vi "CF_FP_to_DSC.vi"(8 "error in (no error)":errorcluster, 10 "str":string[](array[string]), 11 "dbl":dbl[](array[numeric])) -> (0 "error out":errorcluster)   [LabVIEW 2016]
panel:
  in  "str var":refnum<k21>[](array[refnum])=["ni.var.psp://housesoftheholy/Leiden CF900/CF_FP_STATE"]
  in  "dbl var":refnum<k21>[](array[refnum])=["ni.var.psp://housesoftheholy/Leiden CF900/Leiden CF FP/CF FP P1", "ni.var.psp://housesoftheholy/Leiden CF900/Leiden CF FP/CF FP P2", "ni.var.psp://housesoftheholy/Leiden CF900/Leiden CF FP/CF FP P3", "ni.var.psp://housesoftheholy/Leiden CF900/Leiden CF FP/CF FP P4", "ni.var.psp://housesoftheholy/Leiden CF900/Leiden CF FP/CF FP P5", "ni.var.psp://housesoftheholy/Leiden CF900/Leiden CF FP/CF FP P6", "ni.var.psp://housesoftheholy/Leiden CF900/Leiden CF FP/CF FP P7", "ni.var.psp://housesoftheholy/Leiden CF900/Leiden CF FP/CF FP Flow", "ni.var.psp://housesoftheholy/Leiden CF900/Leiden CF FP/CF FP MG0", "ni.var.psp://housesoftheholy/Leiden CF900/Leiden CF FP/CF FP MG1", "ni.var.psp://housesoftheholy/Leiden CF900/Leiden CF FP/CF FP MG2", "ni.var.psp://housesoftheholy/Leiden CF900/Leiden CF FP/CF FP MG3", "ni.var.psp://housesoftheholy/Leiden CF900/Leiden CF FP/CF FP MG4", "ni.var.psp://housesoftheholy/Leiden CF900/Leiden CF FP/CF FP MG5", "ni.var.psp://housesoftheholy/Leiden CF900/Leiden CF FP/CF FP PT on", "ni.var.psp://housesoftheholy/Leiden CF900/Leiden CF FP/CF FP W_in", "ni.var.psp://housesoftheholy/Leiden CF900/Leiden CF FP/CF FP W_out", "ni.var.psp://housesoftheholy/Leiden CF900/Leiden CF FP/CF FP He", "ni.var.psp://housesoftheholy/Leiden CF900/Leiden CF FP/CF FP oil", "ni.var.psp://housesoftheholy/Leiden CF900/Leiden CF FP/CF FP P_low", "ni.var.psp://housesoftheholy/Leiden CF900/Leiden CF FP/CF FP P_high", "ni.var.psp://housesoftheholy/Leiden CF900/Leiden CF FP/CF FP PT current", "ni.var.psp://housesoftheholy/Leiden CF900/Leiden CF FP/CF FP state0", "ni.var.psp://housesoftheholy/Leiden CF900/Leiden CF FP/CF FP state1", "ni.var.psp://housesoftheholy/Leiden CF900/Leiden CF FP/CF FP state2"]
  # "CF FP to DSC"
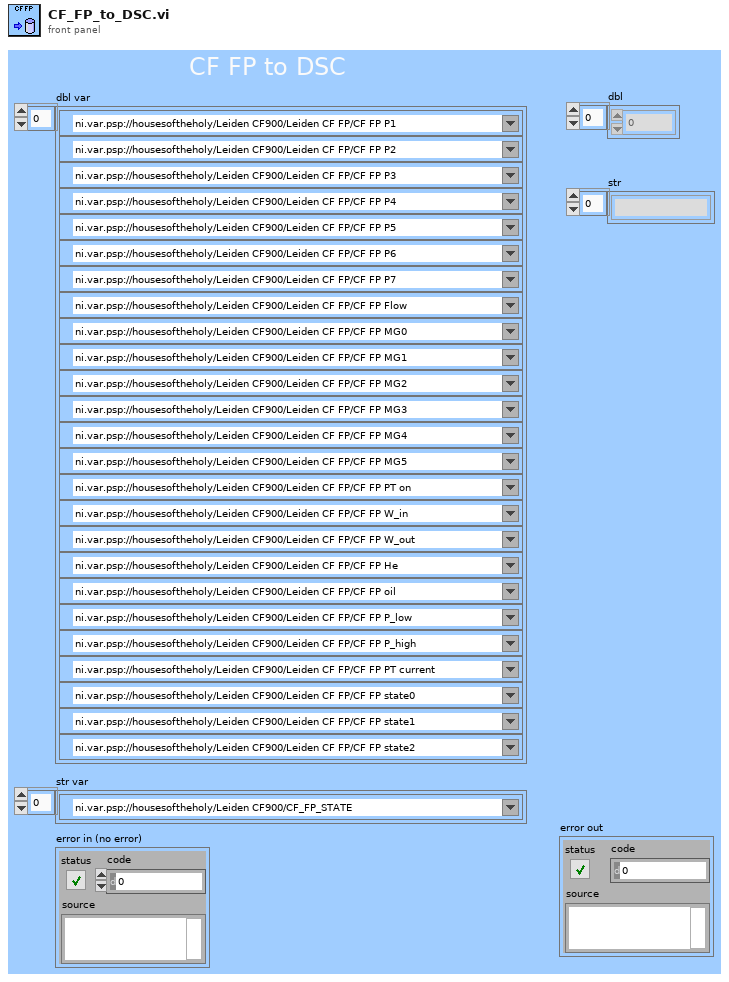
[diagram p1: front panel]
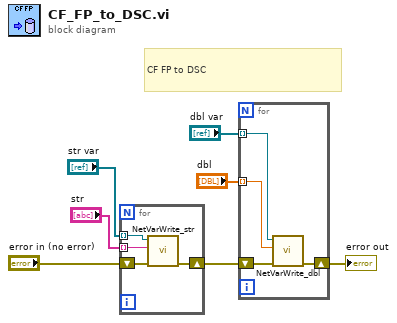
[diagram p0: block diagram]
diagram:
  # "CF FP to DSC"
  n1 = for {
    tunnel: "str var" -> [w8] mode=indexing
    tunnel: "str" -> [w11] mode=indexing
    shift-right: [w9] -> w2
    shift-left: "error in (no error)" -> [w10]
    n2 = call "NetVarWrite_str.vi"("error in (no error)"=w10, "String"=w11, "Refnum in"=w8) -> ("error out"=w9:errorcluster)  [unwired: 8 in]
  }
  n3 = for {
    tunnel: "dbl var" -> [w14] mode=indexing
    tunnel: "dbl" -> [w15] mode=indexing
    shift-right: [w12] -> w1
    shift-left: w2 -> [w13]
    n4 = call "NetVarWrite_dbl.vi"("error in (no error)"=w13, "Numeric"=w15, "Refnum in"=w14) -> ("error out"=w12:errorcluster)  [unwired: 8 in]
  }
  "error out" <- w1
